vi "T564_Numeric(SI)FromSETresponse.vi"(10 "StringIn":string, 11 "Prefix":string) -> (3 "SI_String":string)   [LabVIEW 2013]
uses:
  <vilib>/regexp/Match Regular Expression.xnode
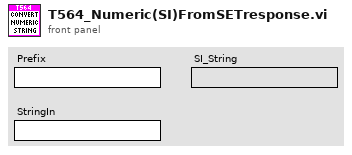
[diagram p1: front panel]
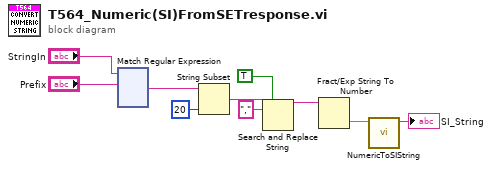
[diagram p0: block diagram]
diagram:
  n1 = xnode "Match Regular Expression"("input string"="StringIn", "regular expression"="Prefix") -> ("after match"=w3:string)  [unwired: 4 in, 4 out]
  n2 = String Subset(string=w3, length (rest)=20 ("length (rest)")) -> (substring=w5:string)  [unwired: 1 in]
  n3 = Search and Replace String(replace all?=TRUE ("replace all? (F)"), input string=w5, search string=",") -> (result string=w8:string)  [unwired: 5 in, 3 out]
  n4 = Fract/Exp String To Number(string=w8) -> (number=w9:dbl)  [unwired: 3 in, 1 out]
  n5 = call "NumericToSIString.vi"("Numeric"=w9) -> ("SI_String"=→"SI_String":string)  [unwired: 9 in, 1 out]
